vi "Initialize.vi"(8 "error in (no error)":errorcluster, 9 "Reset (True)":bool=TRUE, 10 "ID Query (True)":bool=TRUE, 11 "VISA resource name":refnum<visa-resource-name>) -> (0 "error out":errorcluster, 3 "VISA resource name out":refnum<visa-resource-name>)   [LabVIEW 2020, in "Stanford Research SR865.lvlib"]
doc: "Establishes communication with the instrument and optionally performs an instrument identification query and/or an instrument reset. It also places the instrument in a default state needed for other instrument driver operations. Therefore, call this VI before calling other instrument driver VIs for this instrument. Generally, you need to call the <b>Initialize</b> VI only once at the beginning of an application."
uses:
  Stanford Research SR865.lvlib
panel:
  # "(c) 2015 National Instruments.  ALL RIGHTS RESERVED."
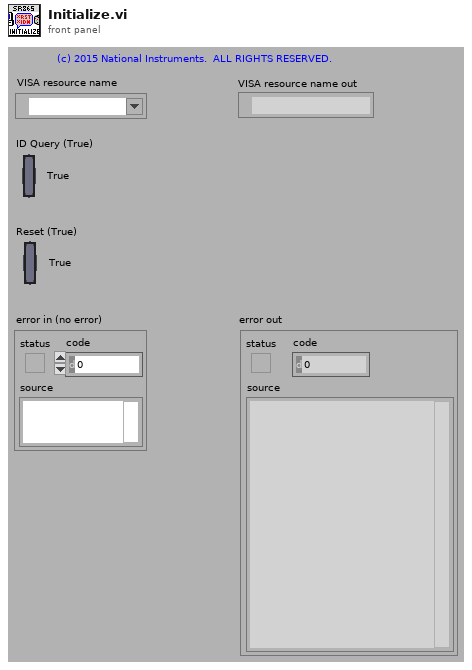
[diagram p1: front panel]
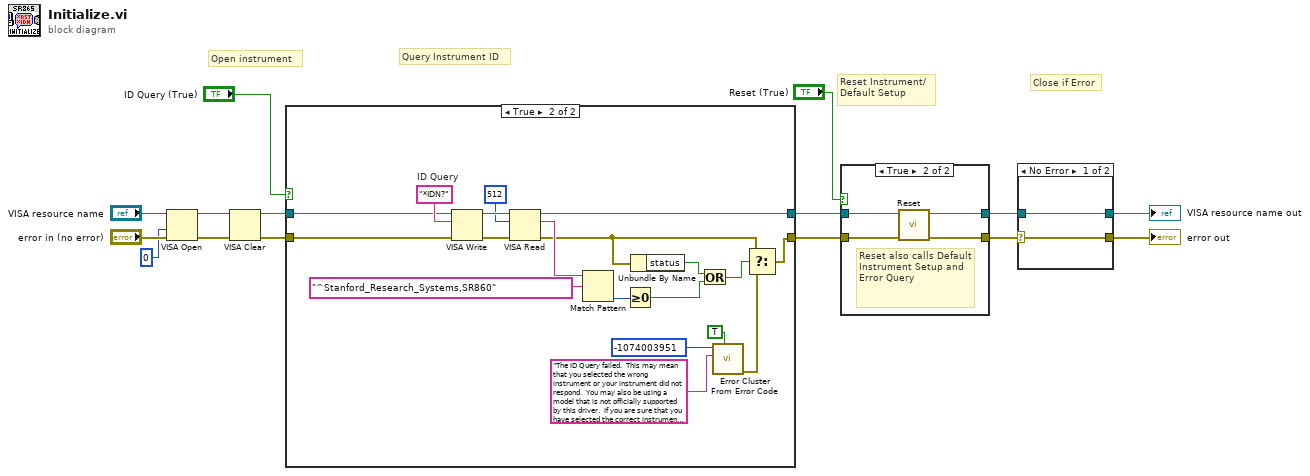
[diagram p0: block diagram]
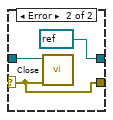
[diagram p2: hidden frame]
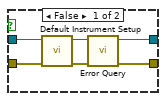
[diagram p3: hidden frame]
diagram:
  # "Close if Error"
  # "Query Instrument ID"
  # "Reset Instrument/\nDefault Setup"
  # "Open instrument"
  n1 = VISA Open(access mode=u32 0, error in (no error)="error in (no error)", VISA resource name="VISA resource name") -> (VISA resource name=w9:refnum<visa-resource-name>, error out=w8:errorcluster)  [unwired: 2 in]
  n2 = VISA Clear(VISA resource name=w9, error in (no error)=w8) -> (VISA resource name out=w3:refnum<visa-resource-name>, error out=w2:errorcluster)
  n3 = case shown="True" "ID Query (True)" {
    tunnel: [w16 w36] -> w15
    tunnel: w3 -> [w17 w19]
    tunnel: w2 -> [w16 w18]
    tunnel: [w17 w35] -> w1
    frame False {
    }
    frame True {
      w29 = "*IDN?"  # ID Query
      n4 = VISA Write(VISA resource name=w19, write buffer=w29, error in (no error)=w18) -> (VISA resource name out=w33:refnum<visa-resource-name>, error out=w32:errorcluster)  [unwired: 1 out]
      n5 = VISA Read(VISA resource name=w33, byte count=u32 512, error in (no error)=w32) -> (VISA resource name out=w35:refnum<visa-resource-name>, read buffer=w34:string, error out=w23:errorcluster)  [unwired: 1 out]
      n6 = Match Pattern(string=w34, regular expression="^Stanford_Research_Systems,SR860") -> (offset past match=w24:i32)  [unwired: 1 in, 3 out]
      n7 = Greater Or Equal To 0?(x=w24) -> (x >= 0?=w21:bool)
      n8 = Unbundle By Name(w23) -> ("status"=w22:bool)
      n9 = Or(x=w22, y=w21) -> (x .or. y?=w20:bool)
      n10 = call <vilib>:"Error Cluster From Error Code.vi"("show call chain? (False)"=TRUE, "error message (\"\")"="The ID Query failed.  This may mean that you selected the wrong instrument or your instrument did not respond.  You may also be using a model that is not officially supported by this driver.  If you are sure that you have selected the correct instrument and it is responding, try disabling the ID Query." ("Source (VI Name)"), "error code (0)"=-1074003951 ("Code")) -> ("error out"=w28:errorcluster)  [unwired: 6 in]
      n11 = Select(t=w23, s=w20, f=w28) -> (s? t:f=w36:errorcluster)
    }
  }
  n12 = case shown="True" "Reset (True)" {
    tunnel: w15 -> [w41 w43]
    tunnel: [w38 w46] -> w4
    tunnel: w1 -> [w42 w44]
    tunnel: [w39 w45] -> w5
    frame False {
      n13 = call "Default Instrument Setup.vi"("error in (no error)"=w41, "VISA resource name"=w42) -> ("error out"=w37:errorcluster, "VISA resource name out"=w40:refnum<visa-resource-name>)  [unwired: 8 in]
      n14 = call "Error Query.vi"("error in (no error)"=w37, "VISA resource name"=w40) -> ("error out"=w38:errorcluster, "VISA resource name out"=w39:refnum<visa-resource-name>)  [unwired: 7 in, 1 out]
    }
    frame True {
      # "Reset also calls Default Instrument Setup and Error Query"
      n15 = call "Reset.vi"("error in (no error)"=w43, "VISA resource name"=w44) -> ("error out"=w46:errorcluster, "VISA resource name out"=w45:refnum<visa-resource-name>)  [unwired: 8 in]
    }
  }
  n16 = case shown="No Error" w4 {
    selector: w4 -> [w47 w49]
    tunnel: w5 -> [w48 w51]
    tunnel: [w48 refnum<visa-resource-name> refnum ("VISA resource name out")] -> w7
    tunnel: [w47 w49] -> w6
    frame No Error {
    }
    frame Error {
      n17 = call "Close.vi"("error in (no error)"=w49, "VISA resource name"=w51) -> ()  [unwired: 10 in]
    }
  }
  "VISA resource name out" <- w7
  "error out" <- w6
